vi "LWXPS_PositionerMagneticTrackPositionAtHomeGet.vi"(0 "XPS Reference IN":refnum<k24>, 2 "Positioner Name":string, 5 "LabVIEW error IN":errorcluster) -> (9 "LabVIEW error OUT":errorcluster, 10 "XPS Reference OUT":refnum<k24>, 11 "XPS Error String":string, 12 "Returned error code":i32, 13 "Res Mod 2 Pi":dbl, 14 "Magnetic track position":dbl, 15 "Reference position":dbl, 16 "Corrected encoder position":dbl, 17 "Phase before calculation":dbl, 18 "Phase after calculation":dbl, 19 "Magnet period":dbl)   [LabVIEW 2014]
uses:
  D:/XPSQ8_LabView_Library/Development/Source/Dll/Newport.XPS.CommandInterface.dll
  Dll/Newport.XPS.CommandInterface.dll
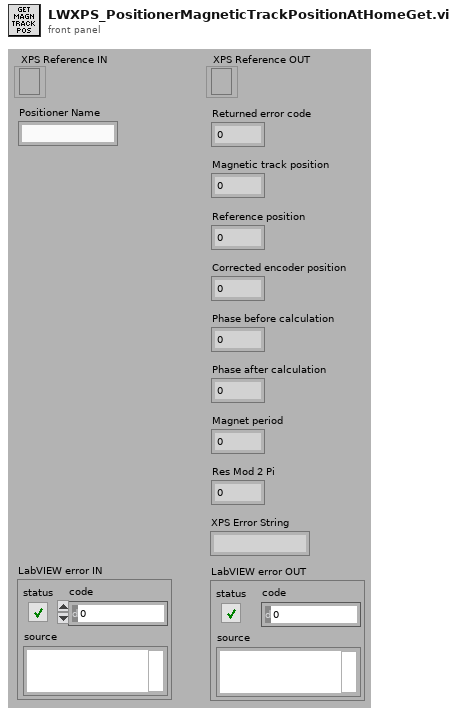
[diagram p1: front panel]
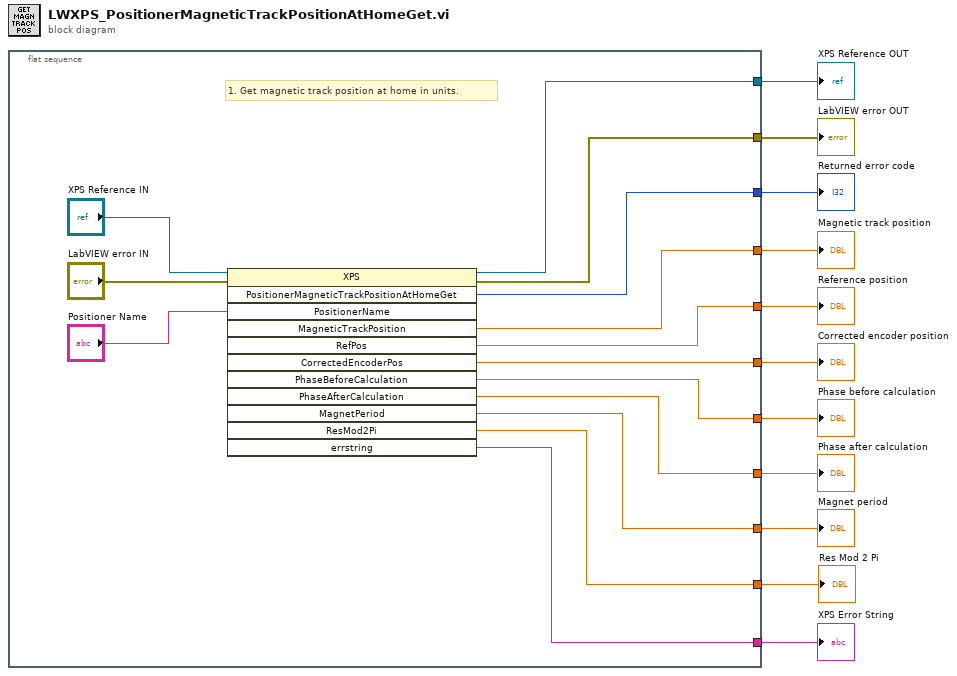
[diagram p0: block diagram]
diagram:
  n1 = flat-sequence {
    tunnel: [w23] -> w11
    tunnel: [w20] -> w10
    tunnel: [w24] -> w9
    tunnel: [w15] -> w3
    tunnel: [w18] -> w8
    tunnel: [w19] -> w5
    tunnel: [w17] -> w7
    tunnel: [w16] -> w6
    tunnel: [w14] -> w4
    tunnel: [w13] -> w1
    tunnel: [w12] -> w2
    frame #0 {
      # "1. Get magnetic track position at home in units."
      n2 = invoke class="XPS" method="PositionerMagneticTrackPositionAtHomeGet"(reference="XPS Reference IN", error in="LabVIEW error IN", "PositionerName"="Positioner Name") -> (reference out=w23:refnum<k24>, error out=w20:errorcluster, "PositionerMagneticTrackPositionAtHomeGet"=w24:i32, "MagneticTrackPosition"=w15:dbl, "RefPos"=w18:dbl, "CorrectedEncoderPos"=w17:dbl, "PhaseBeforeCalculation"=w16:dbl, "PhaseAfterCalculation"=w19:dbl, "MagnetPeriod"=w14:dbl, "ResMod2Pi"=w13:dbl, "errstring"=w12:string)  [unwired: 9 in, 1 out]
    }
  }
  "XPS Error String" <- w2
  "XPS Reference OUT" <- w11
  "LabVIEW error OUT" <- w10
  "Returned error code" <- w9
  "Reference position" <- w8
  "Corrected encoder position" <- w7
  "Phase before calculation" <- w6
  "Phase after calculation" <- w5
  "Magnet period" <- w4
  "Magnetic track position" <- w3
  "Res Mod 2 Pi" <- w1
